vi "reset_devices.vi"(8 "error in (no error)":errorcluster, 11 "ui_input":T1) -> (0 "error out":errorcluster, 3 "UI_out":T1)   [LabVIEW 2017]
uses:
  ui.ctl
  ui_buttons.ctl
  types/boc_type.ctl
  <vilib>/Utility/error.llb/DialogType.ctl
  <instrlib>/Siglent SDG X Series/Siglent SDG X Series.lvlib
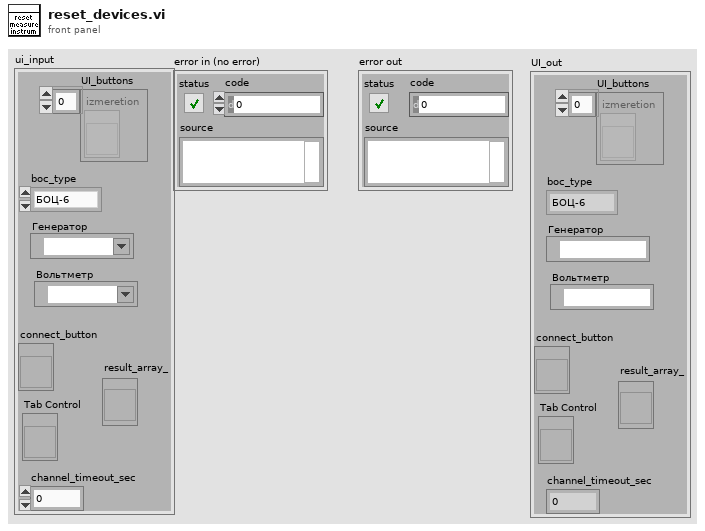
[diagram p1: front panel]
types:
  T1 = typedef "ui.ctl" = cluster{"UI_buttons":T2, "Tab Control":refnum<vi>, "connect_button":refnum<vi>, "generator":refnum<visa-resource-name>, "voltmetr":refnum<visa-resource-name>, "channel_timeout_sec":dbl, "boc_type":T3, "result_array_":refnum<vi>}
  T2 = typedef "ui_buttons.ctl" = refnum<vi>[]
  T3 = typedef "boc_type.ctl" = enum16{"БОЦ-6", "БОЦ-12"}
  T4 = typedef "DialogType.ctl" = u16
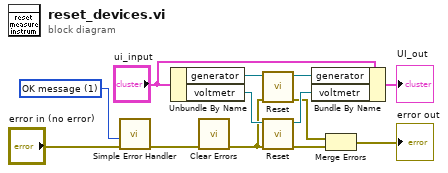
[diagram p0: block diagram]
diagram:
  w7 = T4 1 items=["no dialog", "OK message", "continue or stop message", "OK message + warnings", "continue/stop + warnings"] ("type of dialog (OK msg:1)")
  n1 = call <vilib>:"Simple Error Handler.vi"("type of dialog (OK msg:1)"=w7, "error in (no error)"="error in (no error)") -> ("error out"=w11:errorcluster)  [unwired: 3 in, 4 out]
  n2 = Unbundle By Name("ui_input") -> ("generator"=w13:refnum<visa-resource-name>, "voltmetr"=w12:refnum<visa-resource-name>)
  n3 = call <vilib>:"Clear Errors.vi"("error in (no error)"=w11) -> ("error out"=w9:errorcluster)  [unwired: 5 in, 1 out]
  n4 = call <instrlib>:"Reset.vi"("error in (no error)"=w9, "VISA resource name"=w13) -> ("error out"=w2:errorcluster, "VISA resource name out"=w4:refnum<visa-resource-name>)  [unwired: 8 in]
  n5 = call <instrlib>:"Reset.vi"("error in (no error)"=w9, "VISA resource name"=w12) -> ("error out"=w1:errorcluster, "VISA resource name out"=w3:refnum<visa-resource-name>)  [unwired: 8 in]
  n6 = Bundle By Name(cluster="ui_input", "generator"=w4, "voltmetr"=w3) -> (→"UI_out":T1)
  n7 = Merge Errors(w2, w1) -> (→"error out":errorcluster)
